vi "generate arrays for pockels cell blanking.vi"() -> (3 "Array":dbl[][](array[numeric]))   [LabVIEW 2012]
uses:
  GFG/GFGbooleanGet.vi
  GFG/GFGnumericGet.vi
  GFG/GFG library.lvlib
panel:
  in  "fpga input adapter sampling rate":i32=36000000
  out "number of pockels cell ao samples per line":dbl=65.0
  out "Waveform Graph 2":dbl[][](graph)
  in  "n":i32=-1
  out "size(s)":i32
  out "piezo data":dbl[](graph)
  out "pockels blanking data":dbl[](graph)
  in  "min pockels cell voltage":dbl
  out "number of pcao samples to blank on each side":dbl
  in  "pockels.cell.ao.samples.per.s":dbl=1200000.0
  out "example piezo array":dbl[](graph)
  out "example pockels cell data":dbl[](graph)
  out "Waveform Graph":dbl[][](graph)
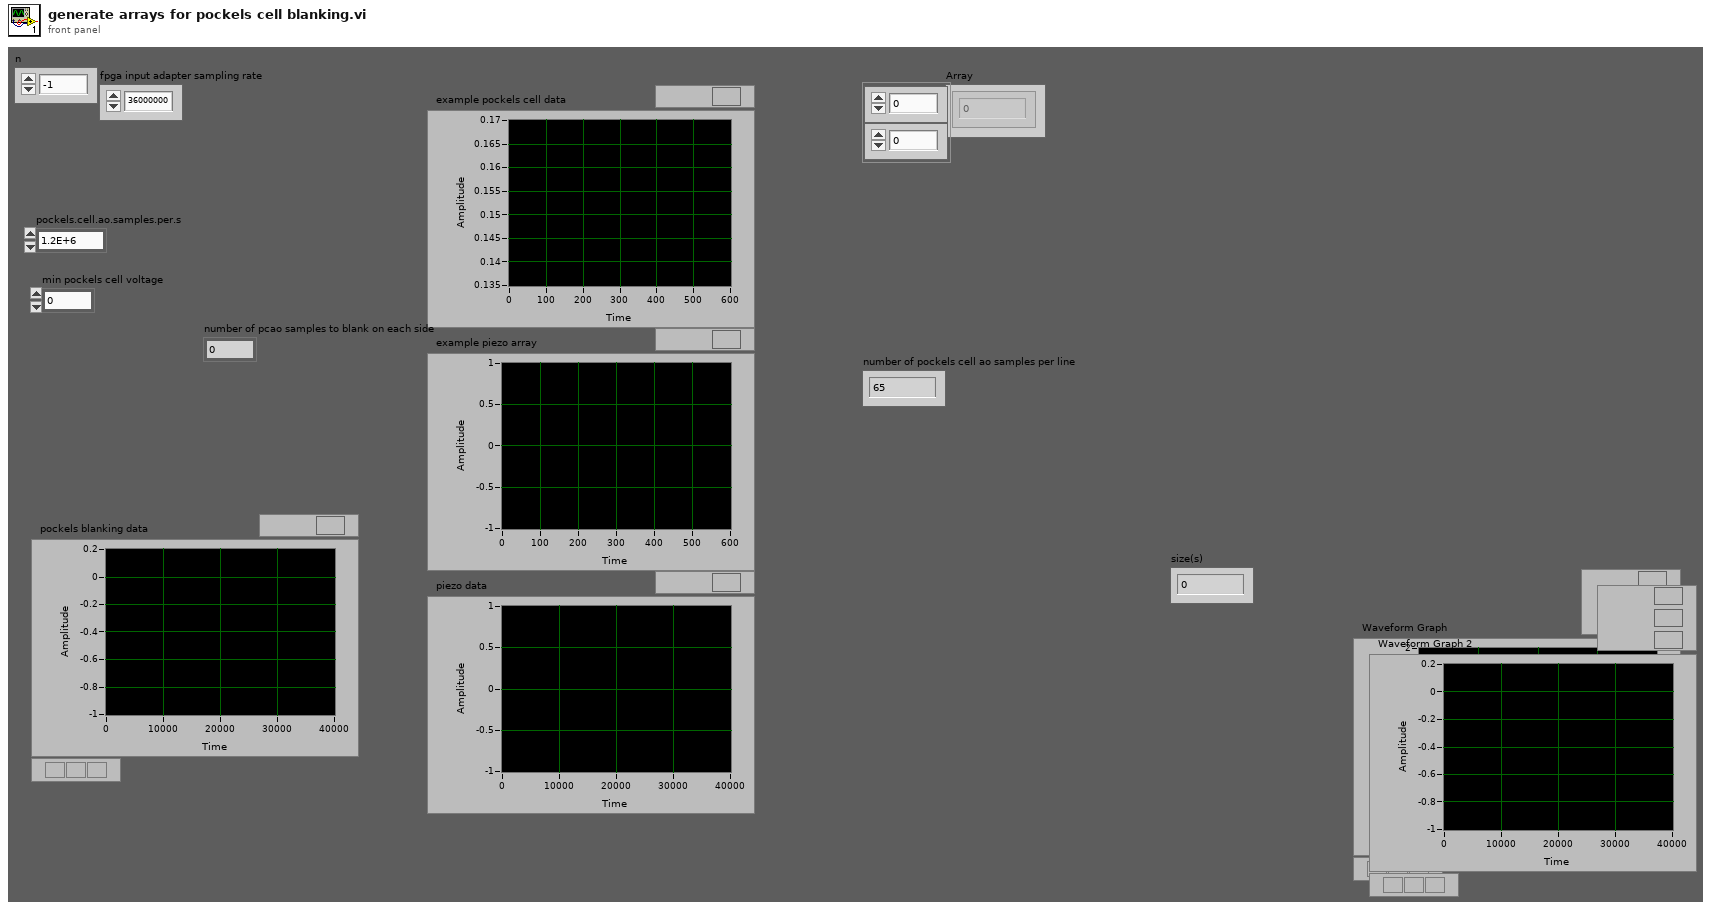
[diagram p1: front panel]
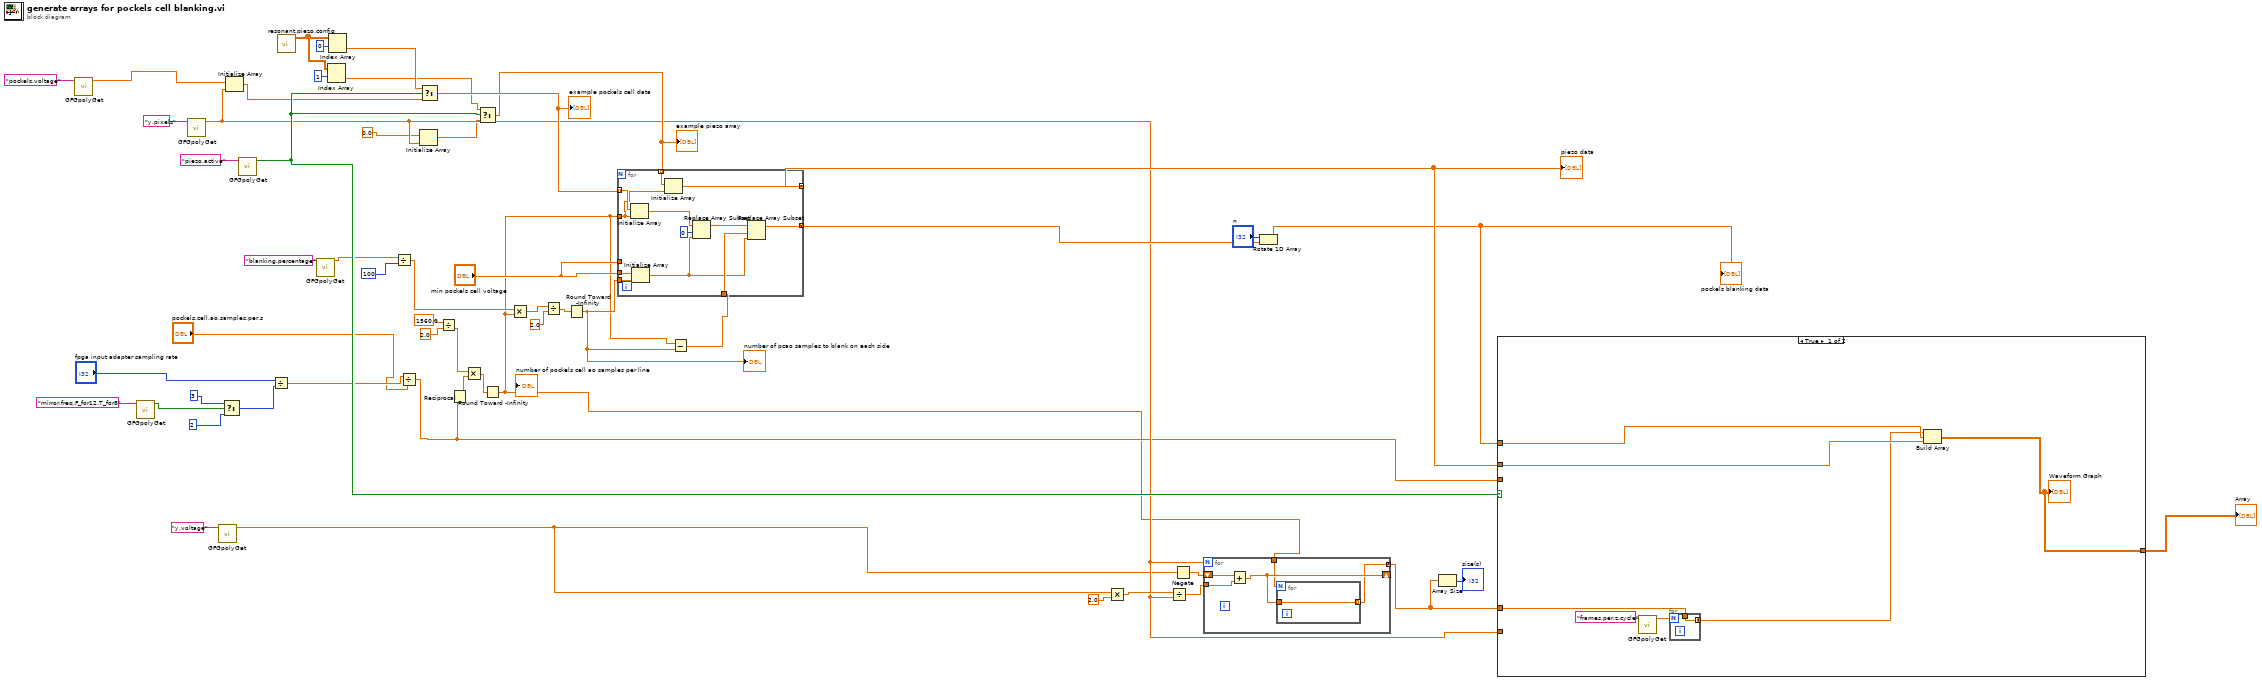
[diagram p0: block diagram]
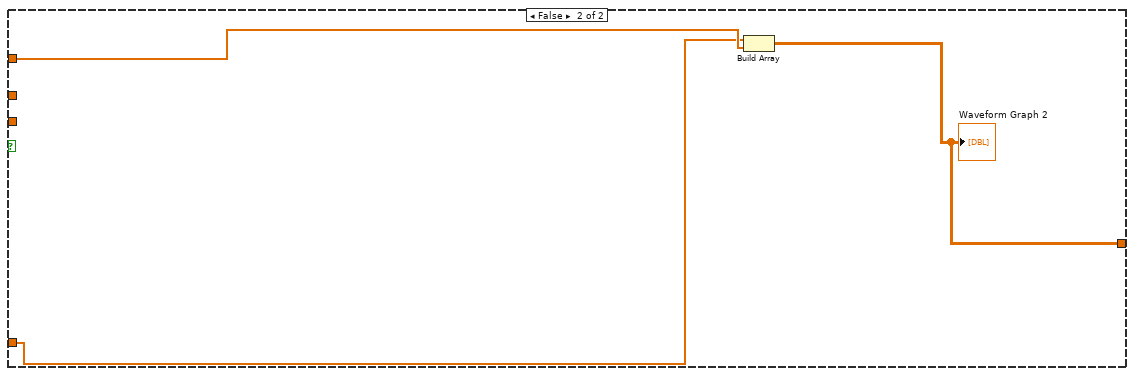
[diagram p2: hidden frame]
diagram:
  n1 = call-poly "GFGpolyGet.vi"("Variable Name in"="pockels.voltage") -> ("Numeric"=w1:dbl)  [unwired: 9 in, 1 out]
  n2 = call-poly "GFGpolyGet.vi"("Variable Name in"="mirror.freq.F_for12.T_for8") -> ("Boolean"=w7:bool)  [unwired: 10 in]
  n3 = call-poly "GFGpolyGet.vi"("Variable Name in"="y.pixels") -> ("Numeric"=w15:dbl)  [unwired: 9 in, 1 out]
  n4 = call-poly "GFGpolyGet.vi"("Variable Name in"="y.voltage" ("Tag in")) -> ("Numeric"=w3:dbl)  [unwired: 9 in, 1 out]
  n5 = Select(t=3, s=w7, f=2) -> (s? t:f=w44:i32)
  n6 = Initialize Array(w1, w15) -> (w16:dbl[])
  n7 = call-poly "GFGpolyGet.vi"("Variable Name in"="piezo.active") -> ("Boolean"=w17:bool)  [unwired: 10 in]
  n8 = Divide(x="fpga input adapter sampling rate", y=w44) -> (x/y=w11:dbl)
  n9 = call "resonant.piezo.config.vi"() -> ("appended array"=w32:dbl[][])  [unwired: 11 in]
  n10 = call-poly "GFGpolyGet.vi"("Variable Name in"="blanking.percentage") -> ("Numeric"=w5:dbl)  [unwired: 9 in, 1 out]
  n11 = Index Array(array=w32, index (row)=1 ("index")) -> (element=w19:dbl[])  [unwired: 1 in]
  n12 = Index Array(array=w32, index (row)=0 ("index")) -> (element=w21:dbl[])  [unwired: 1 in]
  n13 = Divide(x=w5, y=u8 100) -> (x/y=w40:dbl)
  n14 = Divide(x=w11, y="pockels.cell.ao.samples.per.s") -> (x/y=w9:dbl)
  n15 = Initialize Array(0.0 ("element"), w15) -> (w13:dbl[])
  n16 = Select(t=w21, s=w17, f=w16) -> (s? t:f=w20:dbl[])
  "example pockels cell data" <- w20
  n17 = Divide(x=1560.0, y=2.0) -> (x/y=w28:dbl)
  n18 = Reciprocal(x=w9) -> (1/x=w26:dbl)
  n19 = Multiply(x=w28, y=w26) -> (x*y=w41:dbl)
  n20 = Select(t=w19, s=w17, f=w13) -> (s? t:f=w18:dbl[])
  "example piezo array" <- w18
  n21 = Round Toward -Infinity(1:w41) -> (0:w8:dbl)
  "number of pockels cell ao samples per line" <- w8
  n22 = Multiply(x=w40, y=w8) -> (x*y=w39:dbl)
  n23 = Divide(x=w39, y=2.0 ("x")) -> (x/y=w38:dbl)
  n24 = Round Toward -Infinity(1:w38) -> (0:w24:dbl)
  "number of pcao samples to blank on each side" <- w24
  n25 = Subtract(x=w8, y=w24) -> (x-y=w12:dbl)
  n26 = for {
    tunnel: w20 -> [w66] mode=indexing
    tunnel: w8 -> [w60]
    tunnel: w12 -> [w64]
    tunnel: [w55] -> w36 mode=concatenating
    tunnel: w24 -> [w63]
    tunnel: "min pockels cell voltage" -> [w62]
    tunnel: w18 -> [w61] mode=indexing
    tunnel: [w58] -> w35 mode=concatenating
    tunnel: "min pockels cell voltage" -> [_]
    n27 = Initialize Array(w66, w60) -> (w57:dbl[])
    n28 = Initialize Array(w62, w63) -> (w59:dbl[])
    n29 = Initialize Array(w61, w60) -> (w58:dbl[])
    n30 = Replace Array Subset(array=w57, new element=w59, index=0) -> (w56:dbl[])
    n31 = Replace Array Subset(array=w56, new element=w59, index=w64) -> (w55:dbl[])
  }
  "piezo data" <- w35
  n32 = Multiply(x=w3, y=2.0) -> (x*y=w53:dbl)
  n33 = Divide(x=w53, y=w15) -> (x/y=w51:dbl)
  n34 = Negate(x=w3) -> (-x=w52:dbl)
  n35 = for {
    N: w15 -> [_]
    tunnel: w51 -> [w70]
    shift-right: [w69] -> _
    shift-left: w52 -> [w71]
    tunnel: [w68] -> w31 mode=concatenating
    tunnel: w8 -> [w67]
    n36 = Add(x=w71, y=w70) -> (x+y=w69:dbl)
    n37 = for {
      N: w67 -> [_]
      tunnel: w69 -> [w72]
      tunnel: [w72] -> w68 mode=indexing
    }
  }
  n38 = Rotate 1D Array(1:w36, 2:"n") -> (0:w23:dbl[])
  "pockels blanking data" <- w23
  n39 = Array Size(array=w31) -> (size(s)=→"size(s)":i32)
  n40 = case shown="True" w17 {
    tunnel: w31 -> [w78 w81]
    tunnel: w15 -> [_ _]
    tunnel: [w74 w82] -> w50
    tunnel: w23 -> [w77 w83]
    tunnel: w35 -> [w76 _]
    tunnel: w9 -> [_ _]
    frame True {
      n41 = call-poly "GFGpolyGet.vi"("Variable Name in"="frames.per.z.cycle" ("Tag in")) -> ("Numeric"=w73:dbl)  [unwired: 9 in, 1 out]
      n42 = for {
        N: w73 -> [_]
        tunnel: w78 -> [w80]
        tunnel: [w80] -> w75 mode=concatenating
      }
      n43 = Build Array(w75, w77, w76) -> (w74:dbl[][])
      "Waveform Graph" <- w74
    }
    frame False {
      n44 = Build Array(w81, w83) -> (w82:dbl[][])
      "Waveform Graph 2" <- w82
    }
  }
  "Array" <- w50
